vi "Arduino_Thermistor_configure.vi"() -> ()   [LabVIEW 2020]
uses:
  Instrument drivers/Arduino/ctls_and_globals/Arduino tx msg cluster.ctl
panel:
  in  "Channel Name":string
  in  "Self-calibration interval (minutes)":sgl=1.0
  out "Output":dbl
  out "Status comment":string
  in  "Port":refnum<visa-resource-name>="COM18"
  in  "Address":u8=10
  # "Use this vi to configure the ADC self-calibration time interval\nThis value is retained in EEPROM and recalled on power-up."
  # "(255 minutes max.)\nSet 0 for never."
  # "PN 04/02/2014"
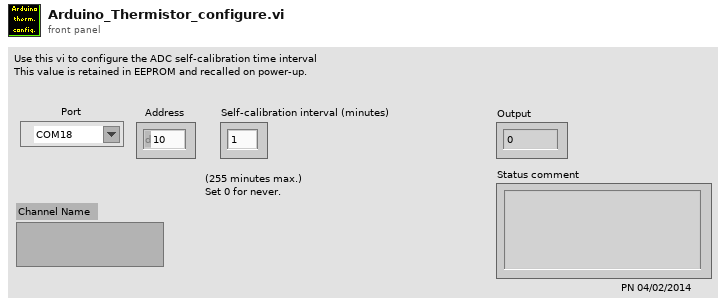
[diagram p1: front panel]
types:
  T1 = typedef "Arduino tx msg cluster.ctl" = cluster{"dest":u8, "A/D/C/I":string, "R/W":string, "chan":u8, "val (float)":sgl}
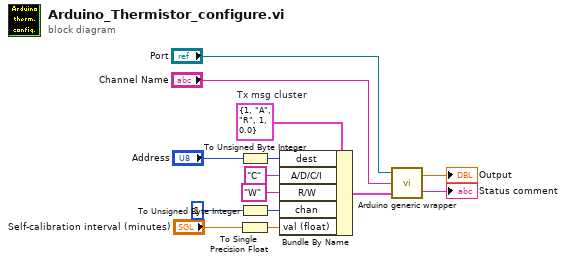
[diagram p0: block diagram]
diagram:
  w10 = T1 {"dest"=1, "A/D/C/I"="A", "R/W"="R", "chan"=1, "val (float)"=0.0}  # Tx msg cluster
  n1 = To Unsigned Byte Integer(number="Address") -> (unsigned 8bit integer=w7:u8)
  n2 = To Unsigned Byte Integer(number=u8 1) -> (unsigned 8bit integer=w3:u8)
  n3 = To Single Precision Float(number="Self-calibration interval (minutes)") -> (single precision float=w12:sgl)
  n4 = Bundle By Name(cluster=w10, "dest"=w7, "A/D/C/I"="C" ("A/D"), "R/W"="W", "chan"=w3, "val (float)"=w12) -> (w9:T1)
  n5 = call "Arduino generic wrapper.vi"("Tx msg cluster"=w9, "Channel Name"="Channel Name", "Port name"="Port") -> ("Scan comment"=→"Status comment":string, "Output"=→"Output":dbl)
